vi "Compute Disparity.vi"(2 "t":cluster{"X":dbl, "Y":dbl}, 3 "r":cluster{"X":dbl, "Y":dbl}, 4 "f":dbl=4.4, 5 "b":dbl=268.0) -> (0 "XYZ (ft)":cluster{"X":dbl, "Y":dbl, "Z":dbl}, 1 "XYZ":cluster{"X":dbl, "Y":dbl, "Z":dbl})   [LabVIEW 2011]
panel:
  out "d":dbl
  # "CamDistOnBot: 268mm"
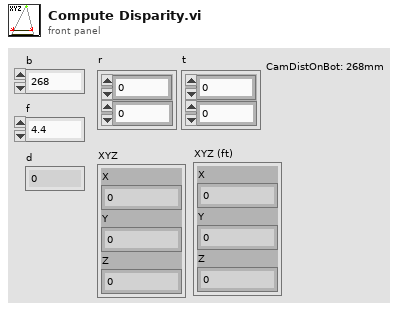
[diagram p1: front panel]
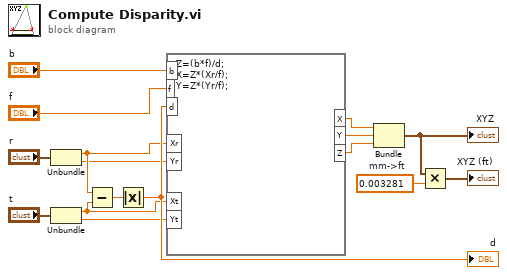
[diagram p0: block diagram]
diagram:
  w10 = 0.003281  # mm->ft
  n1 = Unbundle("r") -> ("X"=w4:dbl, "Y"=w3:dbl)
  n2 = Unbundle("t") -> ("X"=w2:dbl, "Y"=w1:dbl)
  n3 = Subtract(x=w4, y=w2) -> (x-y=w8:dbl)
  n4 = Absolute Value(x=w8) -> (abs(x)=w7:dbl)
  "d" <- w7
  n5 = formula code="Z=(b*f)/d;\nX=Z*(Xr/f);\nY=Z*(Yr/f);"("b"="b", "f"="f", "Xr"=w4, "Xt"=w2, "d"=w7, "Yr"=w3, "Yt"=w1) -> ("Z"=w12:dbl, "X"=w14:dbl, "Y"=w13:dbl)
  n6 = Bundle("X"=w14, "Y"=w13, "Z"=w12) -> (w11:cluster{"X":dbl, "Y":dbl, "Z":dbl})  [unwired: 1 in]
  "XYZ" <- w11
  n7 = Multiply(x=w11, y=w10) -> (x*y=→"XYZ (ft)":cluster{"X":dbl, "Y":dbl, "Z":dbl})
